vi "exportRobotModelData.vi"(5 "RobotModelFolder":string, 6 "triples (V0, Vf, V_sent)":dbl[][](array[numeric]), 7 "CrashCases":T3[](array[typedef]), 8 "error in (no error)":errorcluster, 9 "Samples":dbl, 10 "RobotModelArray":T1, 11 "Game in":refnum<class "Game.lvclass">) -> (0 "error out":errorcluster, 1 "mean":dbl[][](array[numeric]), 2 "Mean":T2[](array[typedef]), 3 "Game out":refnum<class "Game.lvclass">)   [LabVIEW 2023, in "Game.lvclass"]
uses:
  Game.lvclass
  Controls/RobotModel.ctl
  Controls/RobotModelTestCrashCase.ctl
  VelocityPlanningTest/Controls/robotModelArray.ctl
  Utilities_class/Utilities.lvclass
panel:
  in  "all_samples_header (default)":string[](array[string])=["V0", "Vf", "V_sent", "D", "dt", "triple_id", "sample_id"]
  in  "generated_triples_header (default)":string[](array[string])=["V0", "Vf", "V_sent"]
  in  "crash_cases_header (default)":string[](array[string])=["ideal_V0", "real_V0", "ideal_Vf", "real_Vf", "V_sent", "est_vel"]
  in  "mean_values_header (default)":string[](array[string])=["V0", "Vf", "V_sent", "D", "dt", "triple_id", "considered_samples"]
  out "STD":T2[](array[typedef])
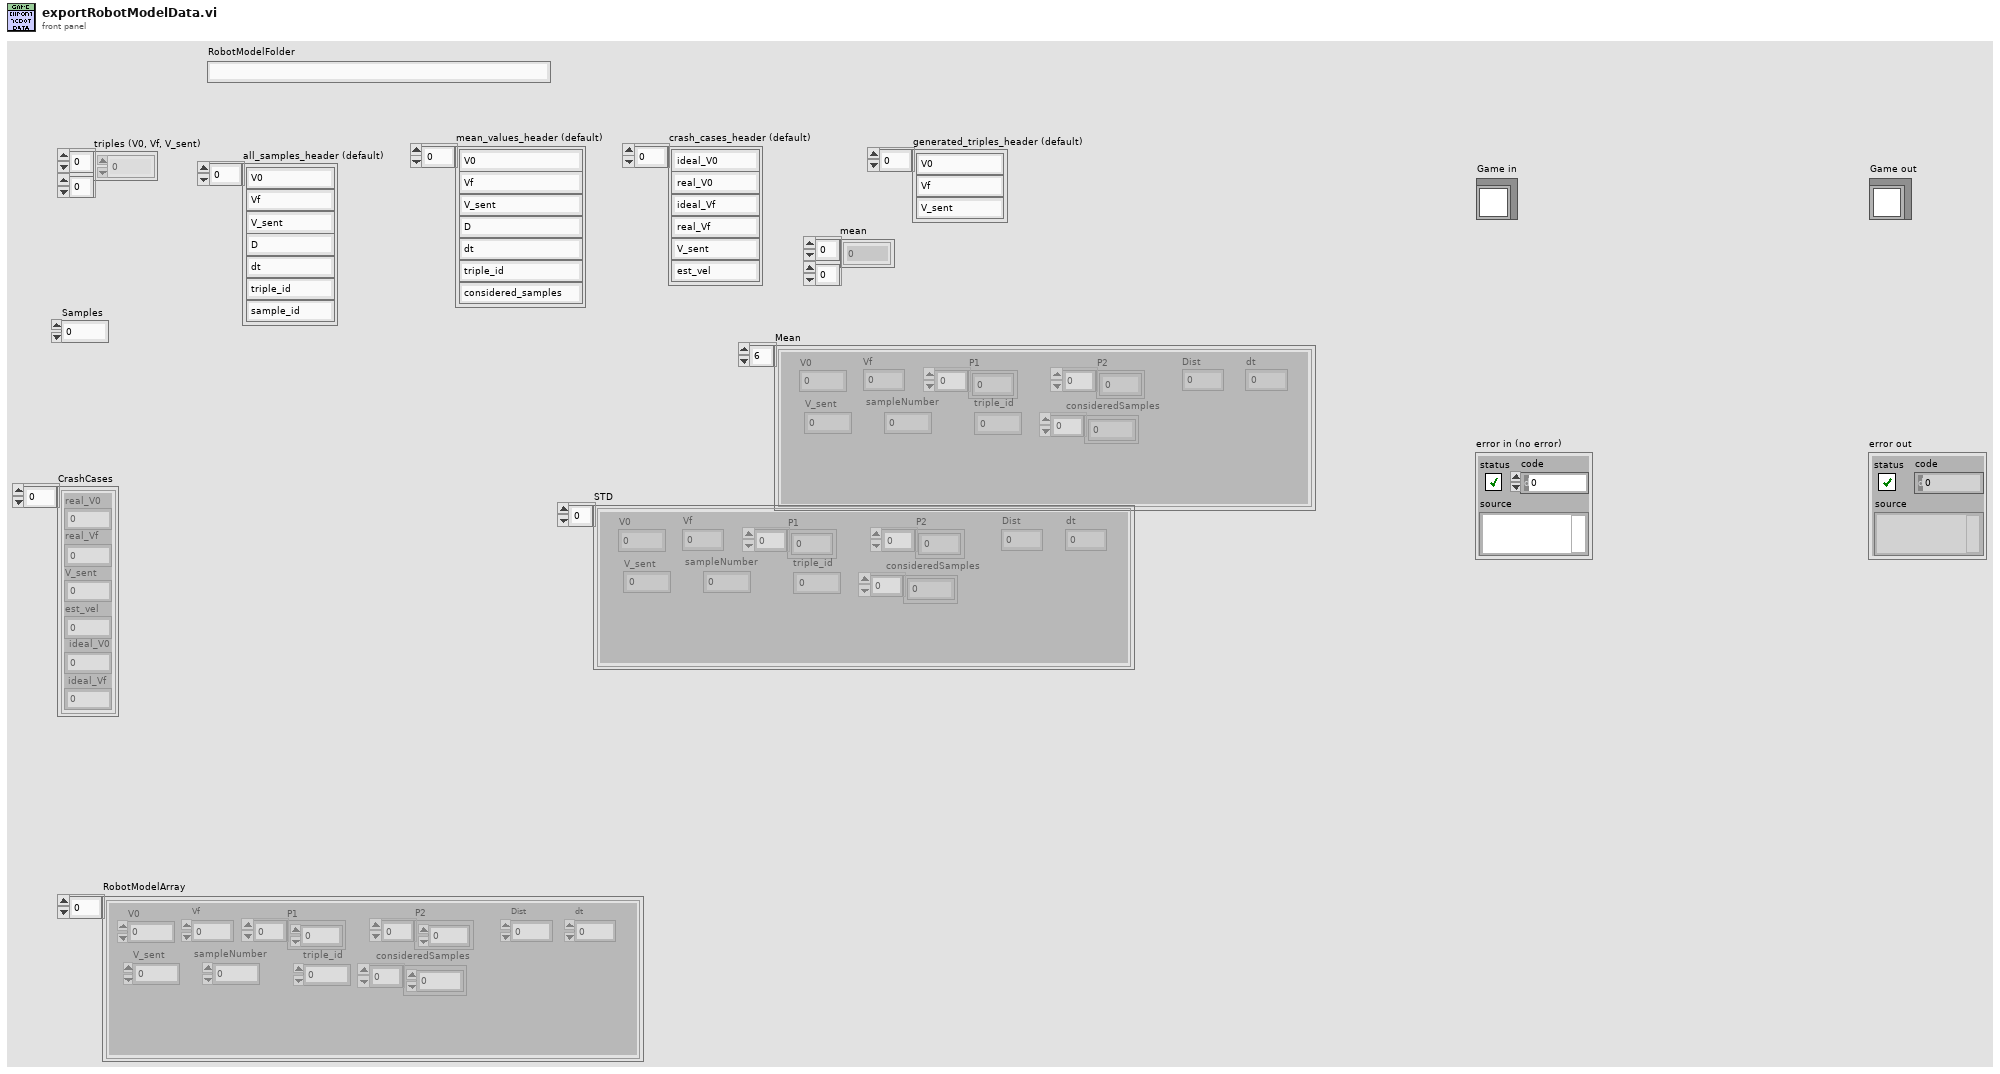
[diagram p1: front panel]
types:
  T1 = typedef "robotModelArray.ctl" = T2[]
  T2 = typedef "RobotModel.ctl" = cluster{"V0":dbl, "Vf":dbl, "Dist":dbl, "dt":dbl, "P1":dbl[], "P2":dbl[], "V_sent":dbl, "sampleNumber":i32, "triple_id":i32, "consideredSamples":dbl[]}
  T3 = typedef "RobotModelTestCrashCase.ctl" = cluster{"real_V0":dbl, "real_Vf":dbl, "V_sent":dbl, "est_vel":dbl, "ideal_V0":dbl, "ideal_Vf":dbl}
  T4 = cluster{"V0":dbl, "Vf":dbl, "Dist":dbl, "dt":dbl, "P1":dbl[], "P2":dbl[], "V_sent":dbl, "sampleNumber":dbl, "triple_id":dbl, "consideredSamples":dbl[]}[]
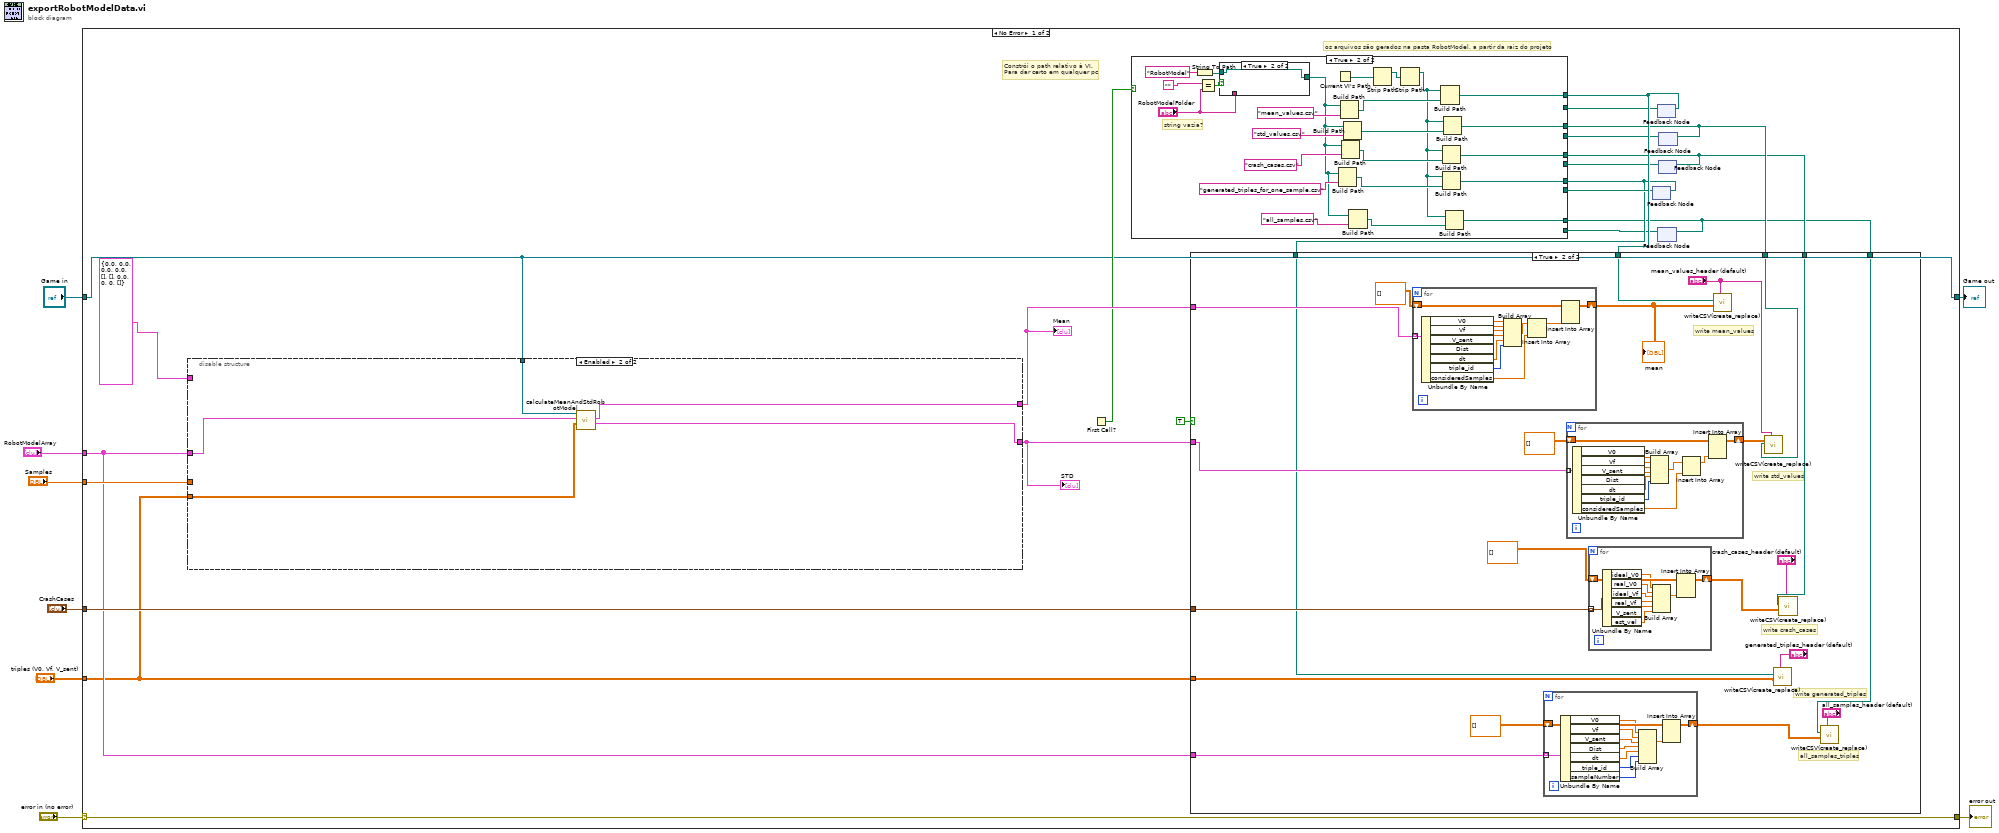
[diagram p0: block diagram]
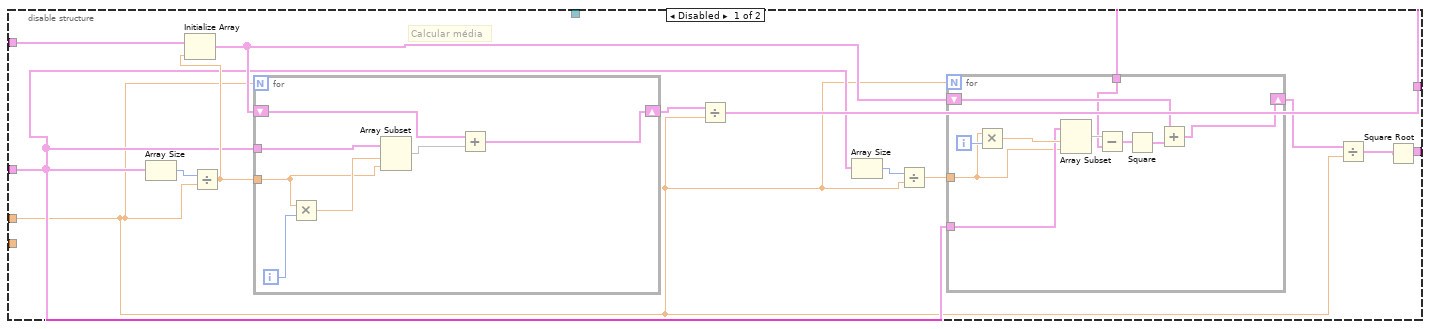
[diagram p2: hidden frame]
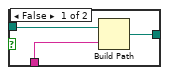
[diagram p4: hidden frame]
diagram:
  n1 = case shown="No Error" "error in (no error)" {
    selector: "error in (no error)" -> [w29 w166]
    tunnel: [w29 w166] -> w7
    tunnel: [w14 w165] -> w5
    tunnel: "Game in" -> [w14 w165]
    tunnel: "RobotModelArray" -> [w13 _]
    tunnel: "Samples" -> [w26 _]
    tunnel: "CrashCases" -> [w24 _]
    tunnel: "triples (V0, Vf, V_sent)" -> [w10 _]
    frame No Error {
      # "os arquivos são gerados na pasta RobotModel, a partir da raiz do projeto"
      # "Constrói o path relativo à VI.\nPara dar certo em qualquer pc"
      n2 = disable-structure shown="Enabled" {
        disable-tunnel: [w42 w64] -> w28
        disable-tunnel: [w41 w63] -> w27
        disable-tunnel: w13 -> [w32 w61]
        disable-tunnel: w26 -> [w31 _]
        disable-tunnel: T2 {"V0"=0.0, "Vf"=0.0, "Dist"=0.0, "dt"=0.0, "P1"=[], "P2"=[], "V_sent"=0.0, "sampleNumber"=0, "triple_id"=0, "consideredSamples"=[]} ("Robot Model") -> [w30 _]
        disable-tunnel: w14 -> [_ w62]
        disable-tunnel: w10 -> [_ w60]
        frame Disabled {
          # "Calcular média"
          n3 = Array Size(array=w32) -> (size(s)=w40:i32)
          n4 = Divide(x=w40, y=w31) -> (x/y=w38:dbl)
          n5 = Initialize Array(w30, w38) -> (w37:T2[])
          n6 = for {
            N: w31 -> [_]
            tunnel: w32 -> [w59]
            tunnel: w38 -> [w56]
            shift-right: [w53] -> w39
            shift-left: w37 -> [w54]
            i -> [w58]
            n7 = Multiply(x=w56, y=w58) -> (x*y=w57:dbl)
            n8 = Array Subset(array=w59, index=w57, length=w56) -> (w55:T1)
            n9 = Add(x=w54, y=w55) -> (x+y=w53:T2[])
          }
          n10 = Divide(x=w39, y=w31) -> (x/y=w42:T4)
          n11 = Array Size(array=w32) -> (size(s)=w36:i32)
          n12 = Divide(x=w36, y=w31) -> (x/y=w35:dbl)
          n13 = for {
            N: w31 -> [_]
            tunnel: w32 -> [w49]
            tunnel: w35 -> [w47]
            shift-right: [w50] -> w34
            shift-left: w37 -> [w51]
            tunnel: w42 -> [w45]
            i -> [w48]
            n14 = Multiply(x=w47, y=w48) -> (x*y=w52:dbl)
            n15 = Array Subset(array=w49, index=w52, length=w47) -> (w46:T1)
            n16 = Subtract(x=w46, y=w45) -> (x-y=w44:T4)
            n17 = Square(x=w44) -> (x^2=w43:T4)
            n18 = Add(x=w51, y=w43) -> (x+y=w50:T4)
          }
          n19 = Divide(x=w34, y=w31) -> (x/y=w33:T4)
          n20 = Square Root(x=w33) -> (sqrt(x)=w41:T4)
        }
        frame Enabled {
          n21 = call "calculateMeanAndStdRobotModel.vi"("triples (V0, Vf, V_sent, id)"=w60, "RobotModelArray"=w61, "Game in"=w62) -> ("Std"=w63:T2[], "Mean"=w64:T2[])  [unwired: 5 in, 2 out]
        }
      }
      "Mean" <- w28
      "STD" <- w27
      n22 = First Call?() -> (First Call?: T/F=w16:bool)
      n23 = feedback #1() -> (w17:path)  [unwired: 1 in]
      n24 = feedback #2() -> (w22:path)  [unwired: 1 in]
      n25 = feedback #3() -> (w11:path)  [unwired: 1 in]
      n26 = feedback #4() -> (w18:path)  [unwired: 1 in]
      n27 = feedback #5() -> (w19:path)  [unwired: 1 in]
      n28 = case shown="True" w16 {
        tunnel: [w68 w91] -> w21
        tunnel: [w67 w90] -> w20
        tunnel: [w69 w89] -> w23
        tunnel: w22 -> [w69 _]
        tunnel: w19 -> [w68 _]
        tunnel: w18 -> [w67 _]
        tunnel: [w66 w88] -> w15
        tunnel: w17 -> [w66 _]
        tunnel: [w65 w70] -> w12
        tunnel: w11 -> [w65 _]
        frame False {
          # "só precisa calcular o path na 1° iteração"
        }
        frame True {
          # "string vazia?"
          n29 = String To Path(string="RobotModel" ("name or relative path")) -> (path=w75:path)
          n30 = Equal?(x="", y="RobotModelFolder") -> (x = y?=w79:bool)
          n31 = case shown="True" w79 {
            tunnel: "RobotModelFolder" -> [w96 _]
            tunnel: [w95 w97] -> w74
            tunnel: w75 -> [w94 w97]
            frame False {
              n32 = Build Path(base path=w94, name or relative path=w96) -> (appended path=w95:path)
            }
            frame True {
            }
          }
          n33 = Current VI's Path() -> (path=w93:path)
          n34 = Build Path(base path=w74, name or relative path="generated_triples_for_one_sample.csv") -> (appended path=w80:path)
          n35 = Build Path(base path=w74, name or relative path="mean_values.csv") -> (appended path=w83:path)
          n36 = Build Path(base path=w74, name or relative path="crash_cases.csv") -> (appended path=w81:path)
          n37 = Build Path(base path=w74, name or relative path="std_values.csv") -> (appended path=w82:path)
          n38 = Build Path(base path=w74, name or relative path="all_samples.csv") -> (appended path=w72:path)
          n39 = Strip Path(path=w93) -> (stripped path=w92:path)  [unwired: 1 out]
          n40 = Strip Path(path=w92) -> (stripped path=w71:path)  [unwired: 1 out]
          n41 = Build Path(base path=w71, name or relative path=w83) -> (appended path=w89:path)
          n42 = Build Path(base path=w71, name or relative path=w81) -> (appended path=w90:path)
          n43 = Build Path(base path=w71, name or relative path=w80) -> (appended path=w88:path)
          n44 = Build Path(base path=w71, name or relative path=w82) -> (appended path=w91:path)
          n45 = Build Path(base path=w71, name or relative path=w72) -> (appended path=w70:path)
        }
      }
      n46 = case shown="True" TRUE {
        tunnel: w28 -> [_ w119]
        tunnel: w27 -> [_ w118]
        tunnel: w21 -> [_ w113]
        tunnel: w20 -> [_ w112]
        tunnel: w24 -> [_ w110]
        tunnel: w23 -> [_ w108]
        tunnel: w10 -> [_ w107]
        tunnel: w15 -> [_ w106]
        tunnel: w13 -> [_ w100]
        tunnel: w12 -> [_ w98]
        frame False {
        }
        frame True {
          # "all_samples_triples"
          # "write generated_triples"
          # "write crash_cases"
          # "write std_values"
          # "write mean_values"
          n47 = for {
            tunnel: w119 -> [w164] mode=indexing
            shift-right: [w162] -> w116
            shift-left: dbl[][] [] ("Array") -> [w163]
            n48 = Unbundle By Name(w164) -> ("V0"=w161:dbl, "Vf"=w160:dbl, "V_sent"=w159:dbl, "Dist"=w158:dbl, "dt"=w157:dbl, "triple_id"=w156:i32, "consideredSamples"=w154:dbl[])
            n49 = Build Array(w161, w160, w159, w158, w157, w156) -> (w155:dbl[])
            n50 = Insert Into Array(array=w155, new element=w154) -> (w153:dbl[])  [unwired: 1 in]
            n51 = Insert Into Array(array=w163, new element=w153) -> (w162:dbl[][])  [unwired: 2 in]
          }
          "mean" <- w116
          n52 = for {
            tunnel: w100 -> [w130] mode=indexing
            shift-right: [w128] -> w102
            shift-left: dbl[][] [] ("Array") -> [w129]
            n53 = Unbundle By Name(w130) -> ("V0"=w122:dbl, "Vf"=w121:dbl, "V_sent"=w127:dbl, "Dist"=w126:dbl, "dt"=w125:dbl, "triple_id"=w124:i32, "sampleNumber"=w120:i32)
            n54 = Build Array(w122, w121, w127, w126, w125, w124, w120) -> (w123:dbl[])
            n55 = Insert Into Array(array=w129, new element=w123) -> (w128:dbl[][])  [unwired: 2 in]
          }
          n56 = for {
            tunnel: w118 -> [w152] mode=indexing
            shift-right: [w150] -> w114
            shift-left: dbl[][] [] ("Array") -> [w151]
            n57 = Unbundle By Name(w152) -> ("V0"=w149:dbl, "Vf"=w148:dbl, "V_sent"=w147:dbl, "Dist"=w146:dbl, "dt"=w145:dbl, "triple_id"=w144:i32, "consideredSamples"=w142:dbl[])
            n58 = Build Array(w149, w148, w147, w146, w145, w144) -> (w143:dbl[])
            n59 = Insert Into Array(array=w143, new element=w142) -> (w141:dbl[])  [unwired: 1 in]
            n60 = Insert Into Array(array=w151, new element=w141) -> (w150:dbl[][])  [unwired: 2 in]
          }
          n61 = for {
            tunnel: w110 -> [w140] mode=indexing
            shift-right: [w138] -> w109
            shift-left: dbl[][] [] ("Array") -> [w139]
            n62 = Unbundle By Name(w140) -> ("ideal_V0"=w132:dbl, "real_V0"=w131:dbl, "ideal_Vf"=w137:dbl, "real_Vf"=w136:dbl, "V_sent"=w135:dbl, "est_vel"=w134:dbl)
            n63 = Build Array(w132, w131, w137, w136, w135, w134) -> (w133:dbl[])
            n64 = Insert Into Array(array=w139, new element=w133) -> (w138:dbl[][])  [unwired: 2 in]
          }
          n65 = call "writeCSV(create_replace).vi"("Header"="mean_values_header (default)", "Array"=w116, "file path (use dialog)"=w108) -> ()  [unwired: 7 in, 2 out]
          n66 = call "writeCSV(create_replace).vi"("Header"="mean_values_header (default)", "Array"=w114, "file path (use dialog)"=w113) -> ()  [unwired: 7 in, 2 out]
          n67 = call "writeCSV(create_replace).vi"("Header"="generated_triples_header (default)", "Array"=w107, "file path (use dialog)"=w106) -> ()  [unwired: 7 in, 2 out]
          n68 = call "writeCSV(create_replace).vi"("Header"="crash_cases_header (default)", "Array"=w109, "file path (use dialog)"=w112) -> ()  [unwired: 7 in, 2 out]
          n69 = call "writeCSV(create_replace).vi"("Header"="all_samples_header (default)", "Array"=w102, "file path (use dialog)"=w98) -> ()  [unwired: 7 in, 2 out]
        }
      }
      n70 = feedback-in #1(w15) -> ()
      n71 = feedback-in #2(w23) -> ()
      n72 = feedback-in #3(w12) -> ()
      n73 = feedback-in #4(w20) -> ()
      n74 = feedback-in #5(w21) -> ()
    }
    frame Error {
    }
  }
  "error out" <- w7
  "Game out" <- w5
